vi "iPS_SetParameters.vi"() -> ()   [LabVIEW 2014]
panel:
  out "Reading of Status 2":string
  in  "Set Field (T)":dbl
  out "Reading of Status":string
  in  "Radio Buttons":enum32{"Hold", "ToSet", "To Zero"}(radio)
  in  "Switch Heater":bool
  in  "error in (no error)":errorcluster
  out "error out":errorcluster
  out "Reading of Switch Heater":string
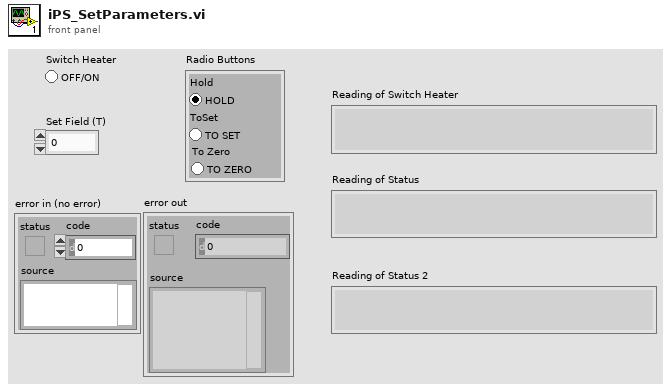
[diagram p1: front panel]
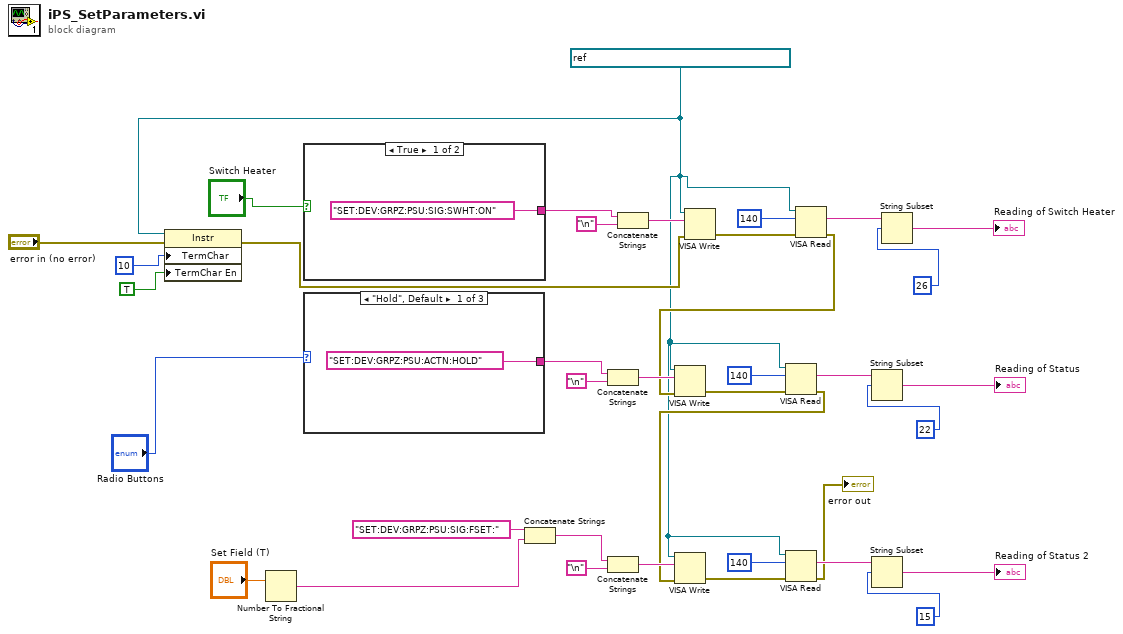
[diagram p0: block diagram]
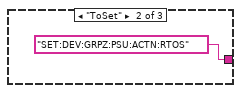
[diagram p2: hidden frame]
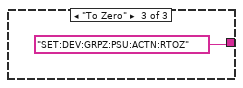
[diagram p3: hidden frame]
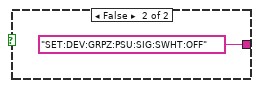
[diagram p4: hidden frame]
diagram:
  w1 = refnum<visa-resource-name> "TCPIP0::192.168.128.3::7020::SOCKET" ("VISA resource name")
  n1 = property class="Instr"(reference=w1, error in="error in (no error)", "TermChar"=10, "TermChar En"=TRUE) -> (error out=w17:errorcluster)  [unwired: 1 out]
  n2 = Number To Fractional String(number="Set Field (T)") -> (F-format string=w12:string)  [unwired: 3 in]
  n3 = case shown="True" "Switch Heater" {
    tunnel: ["SET:DEV:GRPZ:PSU:SIG:SWHT:ON" ("string") "SET:DEV:GRPZ:PSU:SIG:SWHT:OFF" ("string")] -> w20
    frame True {
    }
    frame False {
    }
  }
  n4 = case shown="\"Hold\", Default" "Radio Buttons" {
    tunnel: ["SET:DEV:GRPZ:PSU:ACTN:HOLD" ("string") "SET:DEV:GRPZ:PSU:ACTN:RTOS" ("string") "SET:DEV:GRPZ:PSU:ACTN:RTOZ" ("string")] -> w26
    frame "Hold", Default {
    }
    frame "ToSet" {
    }
    frame "To Zero" {
    }
  }
  n5 = Concatenate Strings("SET:DEV:GRPZ:PSU:SIG:FSET:" ("string"), w12) -> (w4:string)
  n6 = Concatenate Strings(w26, "\n") -> (w27:string)
  n7 = Concatenate Strings(w4, "\n") -> (w6:string)
  n8 = Concatenate Strings(w20, "\n") -> (w21:string)
  n9 = VISA Write(VISA resource name=w1, write buffer=w21, error in (no error)=w17) -> (error out=w25:errorcluster)  [unwired: 2 out]
  n10 = VISA Read(VISA resource name=w1, byte count=140, error in (no error)=w25) -> (read buffer=w22:string, error out=w18:errorcluster)  [unwired: 2 out]
  n11 = VISA Write(VISA resource name=w1, write buffer=w27, error in (no error)=w18) -> (error out=w32:errorcluster)  [unwired: 2 out]
  n12 = VISA Read(VISA resource name=w1, byte count=140, error in (no error)=w32) -> (read buffer=w28:string, error out=w3:errorcluster)  [unwired: 2 out]
  n13 = VISA Write(VISA resource name=w1, write buffer=w6, error in (no error)=w3) -> (error out=w11:errorcluster)  [unwired: 2 out]
  n14 = VISA Read(VISA resource name=w1, byte count=140, error in (no error)=w11) -> (read buffer=w7:string, error out=→"error out":errorcluster)  [unwired: 2 out]
  n15 = String Subset(string=w28, offset (0)=22) -> (substring=→"Reading of Status":string)  [unwired: 1 in]
  n16 = String Subset(string=w7, offset (0)=15) -> (substring=→"Reading of Status 2":string)  [unwired: 1 in]
  n17 = String Subset(string=w22, offset (0)=26) -> (substring=→"Reading of Switch Heater":string)  [unwired: 1 in]
